vi "Get All RC MAX MIN Values.vi"(8 "error in (no error)":errorcluster, 10 "Aircraft ID":u8, 11 "RC Channel":u16) -> (0 "error out":errorcluster)   [LabVIEW 2014]
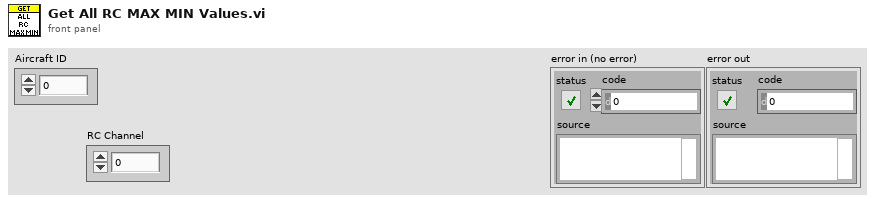
[diagram p1: front panel]
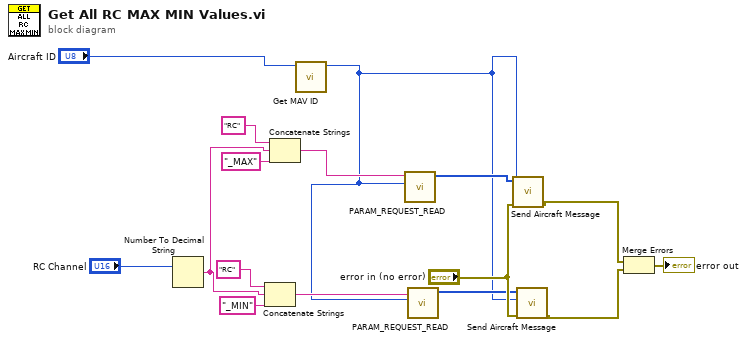
[diagram p0: block diagram]
diagram:
  n1 = Number To Decimal String(number="RC Channel") -> (decimal integer string=w11:string)  [unwired: 1 in]
  n2 = Concatenate Strings("RC" ("string"), w11, "_MIN" ("string")) -> (w10:string)
  n3 = Concatenate Strings("RC" ("string"), w11, "_MAX" ("string")) -> (w12:string)
  n4 = call "Get MAV ID.vi"("Aircraft Index"="Aircraft ID") -> ("Aircraft ID"=w1:u8)  [unwired: 9 in, 1 out]
  n5 = call "PARAM_REQUEST_READ.vi"("Target System and Target Component"=w1, "param_id"=w12) -> ("MAVLink Message"=w6:u8[])  [unwired: 9 in]
  n6 = call "PARAM_REQUEST_READ.vi"("Target System and Target Component"=w1, "param_id"=w10) -> ("MAVLink Message"=w3:u8[])  [unwired: 9 in]
  n7 = call "Send Aircraft Message.vi"("error in (no error)"="error in (no error)", "Aircraft ID"=w1, "MAVLink Message"=w6) -> ("error out"=w7:errorcluster)  [unwired: 8 in]
  n8 = call "Send Aircraft Message.vi"("error in (no error)"="error in (no error)", "Aircraft ID"=w1, "MAVLink Message"=w3) -> ("error out"=w5:errorcluster)  [unwired: 8 in]
  n9 = Merge Errors(w7, w5) -> (→"error out":errorcluster)
